vi "Status Set or Query SESER.vi"(0 "VISA resource name":refnum<visa-resource-name>, 5 "Set/Query (F:Query)":bool, 7 "Sent To Device (CH1-8 F:0)":T1, 11 "error in (no error)":errorcluster) -> (4 "VISA resource name out":refnum<visa-resource-name>, 8 "Read From Device":T1, 15 "error out":errorcluster)   [LabVIEW 2015, in "Chroma ATE 6310.lvlib"]
doc: "This VI sets or queries the bits in the instrument's IEEE-488.2 Standard Event Status Enable register.\n\nWhen you choose \"Set\",you can use the control cluster \"Set To Instrument\" to set the register.And when choosing \"Query\", you can read status from the indicator cluster \"Read From Instrument\"."
uses:
  <instrlib>/Chroma ATE 6310/Chroma ATE 6310.lvlib
panel:
  # "Standard Event Status Enable Register"
  # "Set\n\nQuery"
  # "-           -        CME    EXE     DDE    QYE        -       OPC\n128        64          32        16          8          4        2           1"
  # "-           -        CME    EXE     DDE    QYE        -       OPC\n128        64          32        16          8          4        2           1"
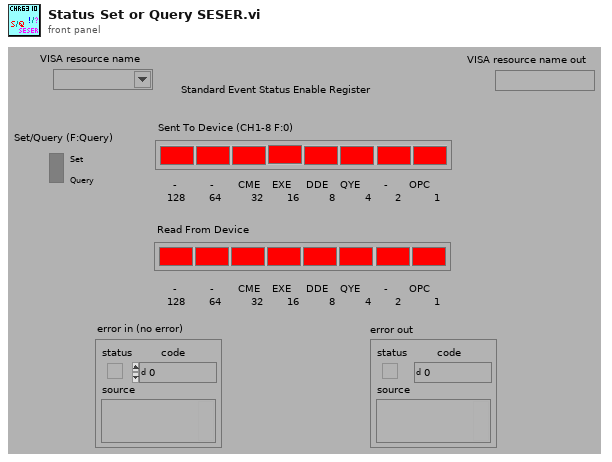
[diagram p1: front panel]
types:
  T1 = cluster{"Bit 7 (F:0)":bool, "Bit 6 (F:0)":bool, "Bit 5 (F:0)":bool, "Bit 4 (F:0)":bool, "Bit 3 (F:0)":bool, "Bit 2 (F:0)":bool, "Bit 1 (F:0)":bool, "Bit 0 (F:0)":bool}
  T2 = cluster{"Bit 7 (F:0)":bool, bool, "Bit 5 (F:0)":bool, "Bit 4 (F:0)":bool, "Bit 3 (F:0)":bool, "Bit 2 (F:0)":bool, bool, bool}
  T3 = cluster{bool, bool, bool, bool, bool, bool, bool, bool}
  T4 = cluster{"[0]":bool, "[1]":bool, "[2]":bool, "[3]":bool, "[4]":bool, "[5]":bool, "[6]":bool, "[7]":bool}
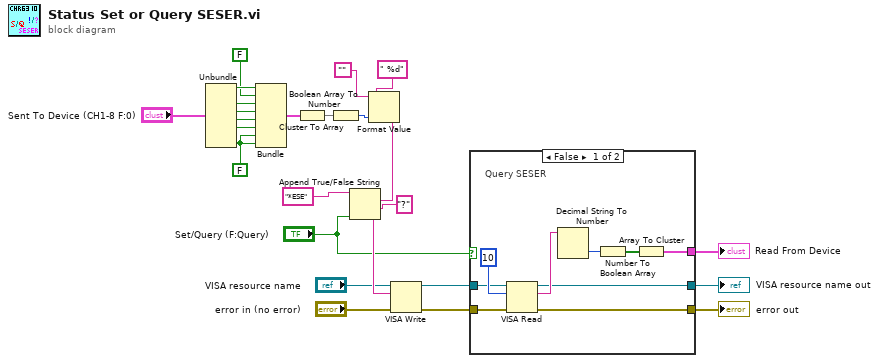
[diagram p0: block diagram]
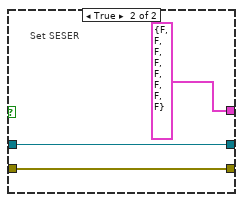
[diagram p2: hidden frame]
diagram:
  w2 = FALSE
  n1 = Unbundle("Sent To Device (CH1-8 F:0)") -> ("Bit 7 (F:0)"=w14:bool, "Bit 5 (F:0)"=w13:bool, "Bit 4 (F:0)"=w12:bool, "Bit 3 (F:0)"=w11:bool, "Bit 2 (F:0)"=w10:bool)  [unwired: 3 out]
  n2 = Bundle("Bit 7 (F:0)"=w14, FALSE, "Bit 5 (F:0)"=w13, "Bit 4 (F:0)"=w12, "Bit 3 (F:0)"=w11, "Bit 2 (F:0)"=w10, w2, w2) -> (w9:T2)  [unwired: 1 in]
  n3 = Cluster To Array(cluster=w9) -> (array=w22:bool[])
  n4 = Boolean Array To Number(Boolean array=w22) -> (number=w21:u32)
  n5 = Format Value(string ("")="", format string=" %d", value (0)=w21) -> (output string=w24:string)
  n6 = Append True/False String(1:"Set/Query (F:Query)", 2:"?", 3:w24, 4:"*ESE") -> (0:w18:string)
  n7 = VISA Write(VISA resource name="VISA resource name", write buffer=w18, error in (no error)="error in (no error)") -> (VISA resource name out=w15:refnum<visa-resource-name>, error out=w16:errorcluster)  [unwired: 1 out]
  n8 = case shown="False" "Set/Query (F:Query)" {
    tunnel: w16 -> [w30 w37]
    tunnel: w15 -> [w31 w36]
    tunnel: [w28 w37] -> w4
    tunnel: [w27 w36] -> w3
    tunnel: [w26 T3 {FALSE, FALSE, FALSE, FALSE, FALSE, FALSE, FALSE, FALSE}] -> w1
    frame False {
      # "Query SESER"
      n9 = VISA Read(VISA resource name=w31, byte count=u32 10, error in (no error)=w30) -> (VISA resource name out=w27:refnum<visa-resource-name>, read buffer=w29:string, error out=w28:errorcluster)  [unwired: 1 out]
      n10 = Decimal String To Number(string=w29) -> (number=w34:i32)  [unwired: 2 in, 1 out]
      n11 = Number To Boolean Array(number=w34) -> (Boolean array=w33:bool[])
      n12 = Array To Cluster(array=w33) -> (cluster=w26:T4)
    }
    frame True {
      # "Set SESER"
    }
  }
  "error out" <- w4
  "VISA resource name out" <- w3
  "Read From Device" <- w1
